vi "Interpolate.vi"(7 "Array":dbl[](array[numeric]), 11 "Index":dbl) -> (3 "Value":dbl)   [LabVIEW 2014]
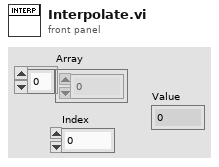
[diagram p1: front panel]
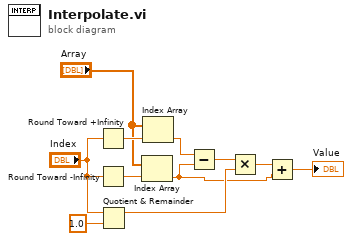
[diagram p0: block diagram]
diagram:
  n1 = Round Toward +Infinity(x="Index") -> (ceil(x): smallest int >= x=w6:dbl)
  n2 = Round Toward -Infinity(1:"Index") -> (0:w5:dbl)
  n3 = Quotient & Remainder(x="Index", y=1.0) -> (x-y*floor(x/y)=w8:dbl)  [unwired: 1 out]
  n4 = Index Array(array="Array", index=w5) -> (element=w2:dbl)
  n5 = Index Array(array="Array", index=w6) -> (element=w3:dbl)
  n6 = Subtract(x=w3, y=w2) -> (x-y=w9:dbl)
  n7 = Multiply(x=w9, y=w8) -> (x*y=w7:dbl)
  n8 = Add(x=w7, y=w2) -> (x+y=→"Value":dbl)
